vi "ALU.vi"(3 "y":bool[](array[boolean])=[FALSE, FALSE, FALSE, FALSE, FALSE, FALSE, FALSE, FALSE, FALSE, FALSE, FALSE, FALSE, FALSE, FALSE, FALSE, FALSE], 4 "x":bool[](array[boolean])=[FALSE, FALSE, FALSE, FALSE, FALSE, FALSE, FALSE, FALSE, FALSE, FALSE, FALSE, FALSE, FALSE, FALSE, FALSE, FALSE], 5 "F":bool[](array[boolean])=[FALSE, FALSE, FALSE, FALSE, FALSE, FALSE]) -> (0 "ng":bool, 1 "zr":bool, 2 "x":bool[](array[boolean]))   [LabVIEW 2012]
doc: "Chip name: ALU\nInputs: x[16], y[16], // Two 16-bit data inputs\nzx, // Zero the x input\nnx, // Negate the x input\nzy, // Zero the y input\nny, // Negate the y input\nf, // Function code: 1 for Add, 0 for And\nno // Negate the out output\nOutputs: out[16], // 16-bit output\nzr, // True iff out=0\nng // True iff out<0\nFunction: if zx then x = 0 // 16-bit zero constant\nif nx then x = !x // Bit-wise negation\nif zy then y = 0 // 16-bit zero constant\nif ny then y = !y // Bit-wise negation\nif f then out = x + y // Integer 2's complement addition\nelse out = x & y // Bit-wise And\nif no then out = !out // Bit-wise negation\nif out=0 then zr = 1 else zr = 0 // 16-bit eq. comparison\nif out<0 then ng = 1 else ng = 0 // 16-bit neg. comparison\nComment: Overflow is neither detected nor handled."
panel:
  # "zx"
  # "nx"
  # "zy"
  # "ny"
  # "f"
  # "no"
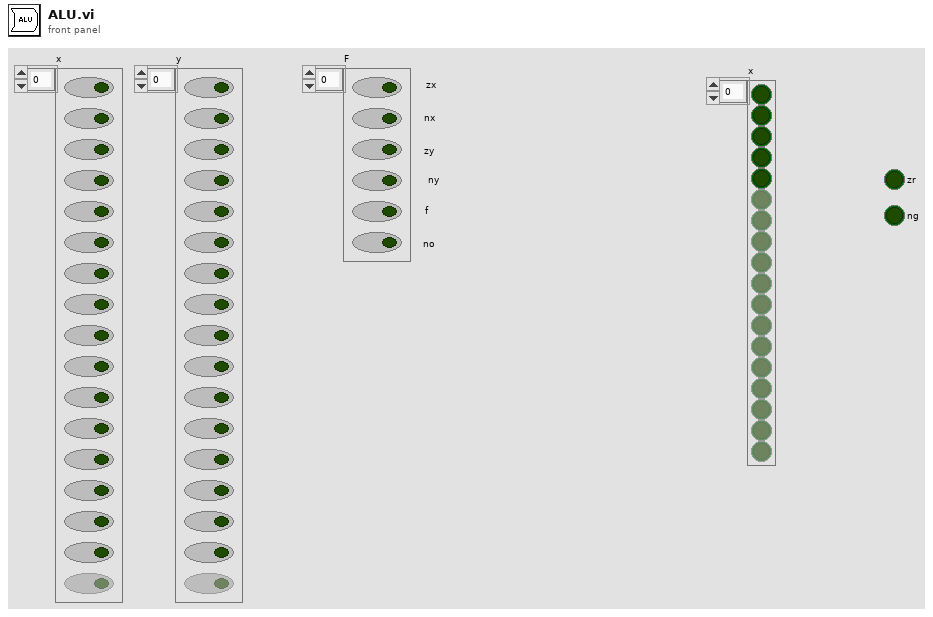
[diagram p1: front panel]
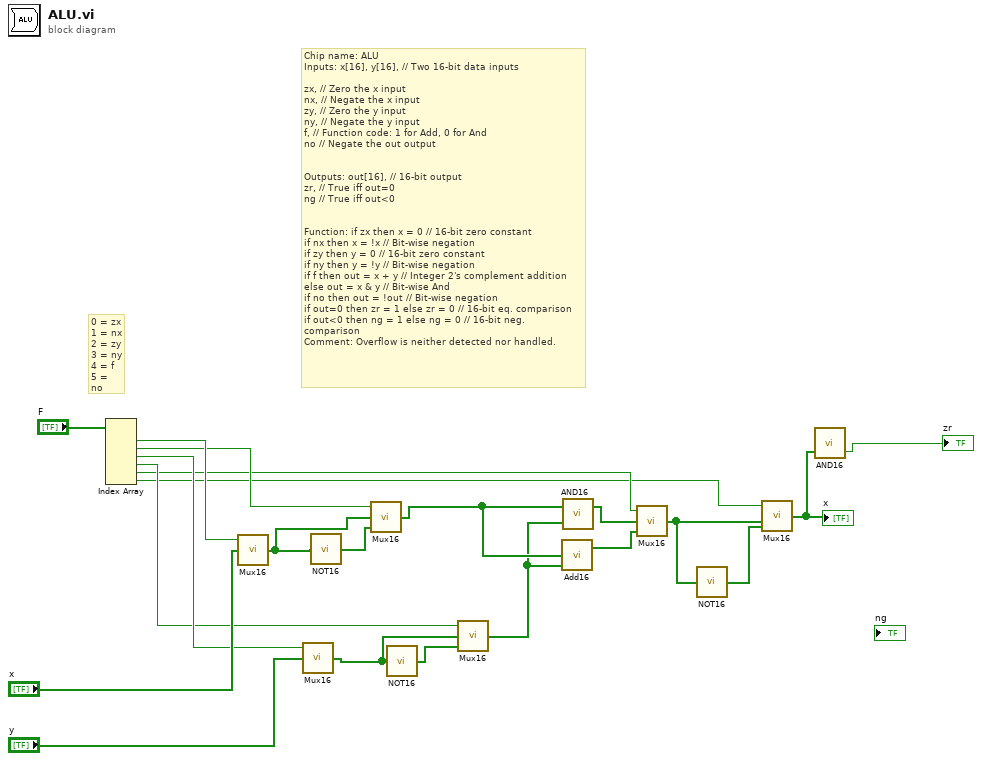
[diagram p0: block diagram]
diagram:
  # "Chip name: ALU\nInputs: x[16], y[16], // Two 16-bit data inputs\n\nzx, // Zero the x input\nnx, // Negate the x input\nzy, // Zero the y input\nny, // Negate the y input\nf, // Function code: 1 for Add, 0 for And\nno // Negate the out output\n\n\nOutputs: out[16], // 16-bit output\nzr, // True iff out=0\nng // True iff out<0\n\n\nFunction: if zx then x = 0 // 16-bit zero constant\nif nx then x = !x // Bit-wise negation\nif zy then y = 0 // 16-bit zero constant\nif ny then y = !y // Bit-wise negation\nif f then out = x + y // Integer 2's complement addition\nelse out = x & y // Bit-wise And\nif no then out = !out // Bit-wise negation\nif out=0 then zr = 1 else zr = 0 // 16-bit eq. comparison\nif out<0 then ng = 1 else ng = 0 // 16-bit neg. comparison\nComment: Overflow is neither detected nor handled."
  # "0 = zx\n1 = nx\n2 = zy\n3 = ny\n4 = f\n5 = no"
  n1 = Index Array(array="F") -> (element #1=w20:bool, element #2=w15:bool, element #3=w14:bool, element #4=w11:bool, element #5=w7:bool, element #6=w5:bool)  [unwired: 6 in]
  n2 = call "Mux16.vi"("A"="x", "s0"=w20) -> ("z"=w16:bool[])  [unwired: 1 in]
  n3 = call "Mux16.vi"("A"="y", "s0"=w14) -> ("z"=w12:bool[])  [unwired: 1 in]
  n4 = call "NOT16.vi"("A"=w16) -> ("z"=w17:bool[])
  n5 = call "Mux16.vi"("B"=w17, "A"=w16, "s0"=w15) -> ("z"=w10:bool[])
  n6 = call "NOT16.vi"("A"=w12) -> ("z"=w13:bool[])
  n7 = call "Mux16.vi"("B"=w13, "A"=w12, "s0"=w11) -> ("z"=w9:bool[])
  n8 = call "Add16.vi"("B"=w9, "A"=w10) -> ("S"=w6:bool[])  [unwired: 1 in, 1 out]
  n9 = call "AND16.vi"("B"=w9, "A"=w10) -> ("z"=w8:bool[])  [unwired: 1 out]
  n10 = call "Mux16.vi"("B"=w6, "A"=w8, "s0"=w7) -> ("z"=w4:bool[])
  n11 = call "NOT16.vi"("A"=w4) -> ("z"=w3:bool[])
  n12 = call "Mux16.vi"("B"=w3, "A"=w4, "s0"=w5) -> ("z"=w2:bool[])
  "x" <- w2
  n13 = call "AND16.vi"("B"=w2) -> ("compound"=→"zr":bool)  [unwired: 1 in, 1 out]
